vi "ReadWrite.ProcessData.Read.vi"(8 "error in (no error)":errorcluster, 10 "timeout ms":i32=100, 11 "ReadWrite in":refnum<class "ReadWrite.lvclass">) -> (0 "error out":errorcluster, 1 "Timeout?":bool, 2 "Values":dbl[](array[numeric]), 3 "ReadWrite out":refnum<class "ReadWrite.lvclass">, 5 "Detect?":bool[](array[boolean]))   [LabVIEW 2015, in "Data Access Engine.lvlib" / "ReadWrite.lvclass"]
uses:
  ReadWrite.lvclass
  ReadWrite.lvclass/ReadWrite.ctl
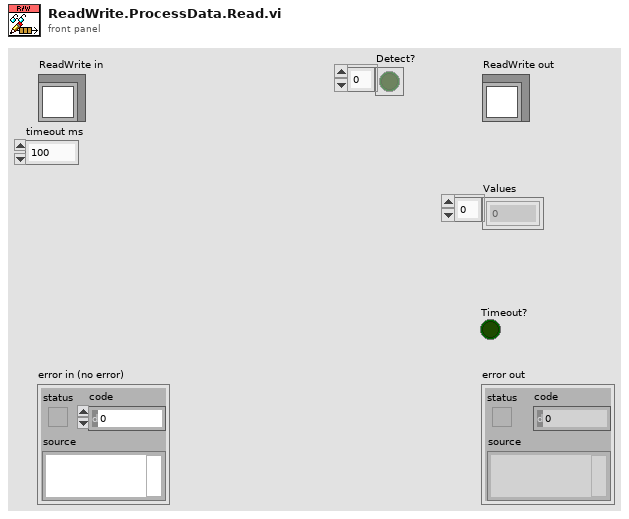
[diagram p1: front panel]
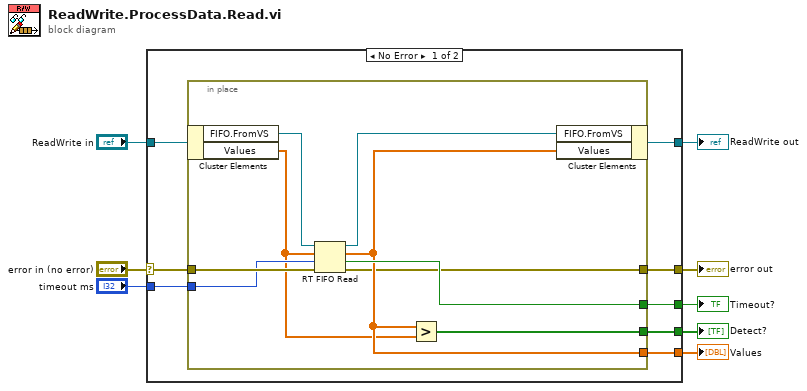
[diagram p0: block diagram]
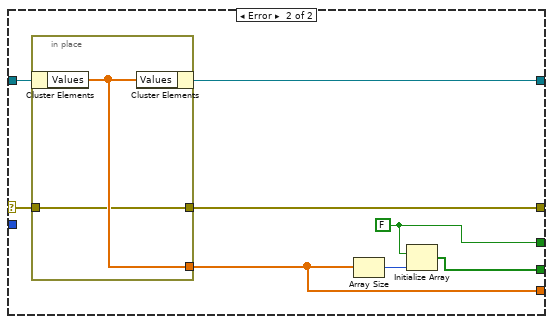
[diagram p2: hidden frame]
diagram:
  n1 = case shown="No Error" "error in (no error)" {
    selector: "error in (no error)" -> [w16 w30]
    tunnel: [w15 w31] -> w7
    tunnel: [w12 w32] -> w5
    tunnel: "ReadWrite in" -> [w13 w33]
    tunnel: [w14 w28] -> w4
    tunnel: "timeout ms" -> [w11 _]
    tunnel: [w10 w26] -> w2
    tunnel: [w9 w27] -> w1
    frame No Error {
      n2 = in-place {
        in-place-border: w16 -> [w24]
        in-place-border: [w17] -> w15
        in-place-border: [w20] -> w14
        in-place-border: w11 -> [w22]
        in-place-border: [w21] -> w10
        in-place-border: [w18] -> w9
        n3 = in-place-cluster #1(w13) -> ("FIFO.FromVS"=w25:refnum<k33>, "Values"=w19:dbl[])
        n4 = RT FIFO Read(0:w25, 1:w19, 2:w22, 3:w24) -> (8:w23:refnum<k33>, 9:w20:dbl[], 10:w21:bool, 11:w17:errorcluster)  [unwired: 1 out]
        n5 = Greater?(x=w20, y=w19) -> (0:w18:bool[])
        n6 = in-place-cluster #1("FIFO.FromVS"=w23, "Values"=w20) -> (w12:refnum<class "ReadWrite.lvclass">)
      }
    }
    frame Error {
      w26 = FALSE ("empty?")
      n7 = in-place {
        in-place-border: [w35] -> w28
        in-place-border: [w34] -> w31
        in-place-border: w30 -> [w34]
        n8 = in-place-cluster #2(w33) -> ("Values"=w35:dbl[])
        n9 = in-place-cluster #2("Values"=w35) -> (w32:refnum<class "ReadWrite.lvclass">)
      }
      n10 = Array Size(array=w28) -> (size(s)=w29:i32)
      n11 = Initialize Array(w26, w29) -> (w27:bool[])
    }
  }
  "error out" <- w7
  "ReadWrite out" <- w5
  "Values" <- w4
  "Timeout?" <- w2
  "Detect?" <- w1
